vi "Conv_Inches_Meters.vi"(10 "INCH":dbl) -> (2 "Meters":dbl)   [LabVIEW 2019, in "Trajectory_Library.lvlib"]
doc: "Convert Inches to Meters"
uses:
  Trajectory_Library.lvlib
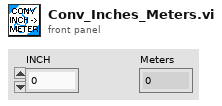
[diagram p1: front panel]
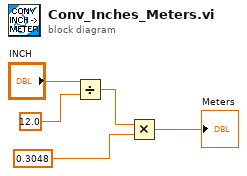
[diagram p0: block diagram]
diagram:
  n1 = Divide(x="INCH", y=12.0) -> (x/y=w1:dbl)
  n2 = Multiply(x=w1, y=0.3048) -> (x*y=→"Meters":dbl)
